vi "Shift_004.vi"() -> ()   [LabVIEW 2019]
panel:
  out "Ep(tk)":dbl[unit][](array[numeric])
  out "Et(tk)":dbl[unit][](array[numeric])
  out "Ek(tk)":dbl[unit][](array[numeric])
  out "Et":cluster{dbl[unit][], dbl[unit][]}(graph)
  out "Ep":cluster{dbl[unit][], dbl[unit][]}(graph)
  out "Ek":cluster{dbl[unit][], dbl[unit][]}(graph)
  out "Et":dbl[unit][](graph)
  out "Ep":dbl[unit][](graph)
  out "Ek":dbl[unit][](graph)
  out "a":cluster{dbl[unit][], dbl[unit][]}(graph)
  out "v":cluster{dbl[unit][], dbl[unit][]}(graph)
  out "x":cluster{dbl[unit][], dbl[unit][]}(graph)
  out "time (tk)":dbl[unit][](array[numeric])
  out "a":dbl[unit][](graph)
  out "v":dbl[unit][](graph)
  out "x":dbl[unit][](graph)
  out "x(tk)":dbl[unit][](array[numeric])
  out "v(tk)":dbl[unit][](array[numeric])
  out "a(k)":dbl[unit][](array[numeric])
  in  "M":dbl[unit]=100.0
  in  "k":dbl[unit]=1000.0
  in  "v0":dbl[unit]
  in  "x0":dbl[unit]=2.0
  in  "Dt":dbl[unit]=1e-05
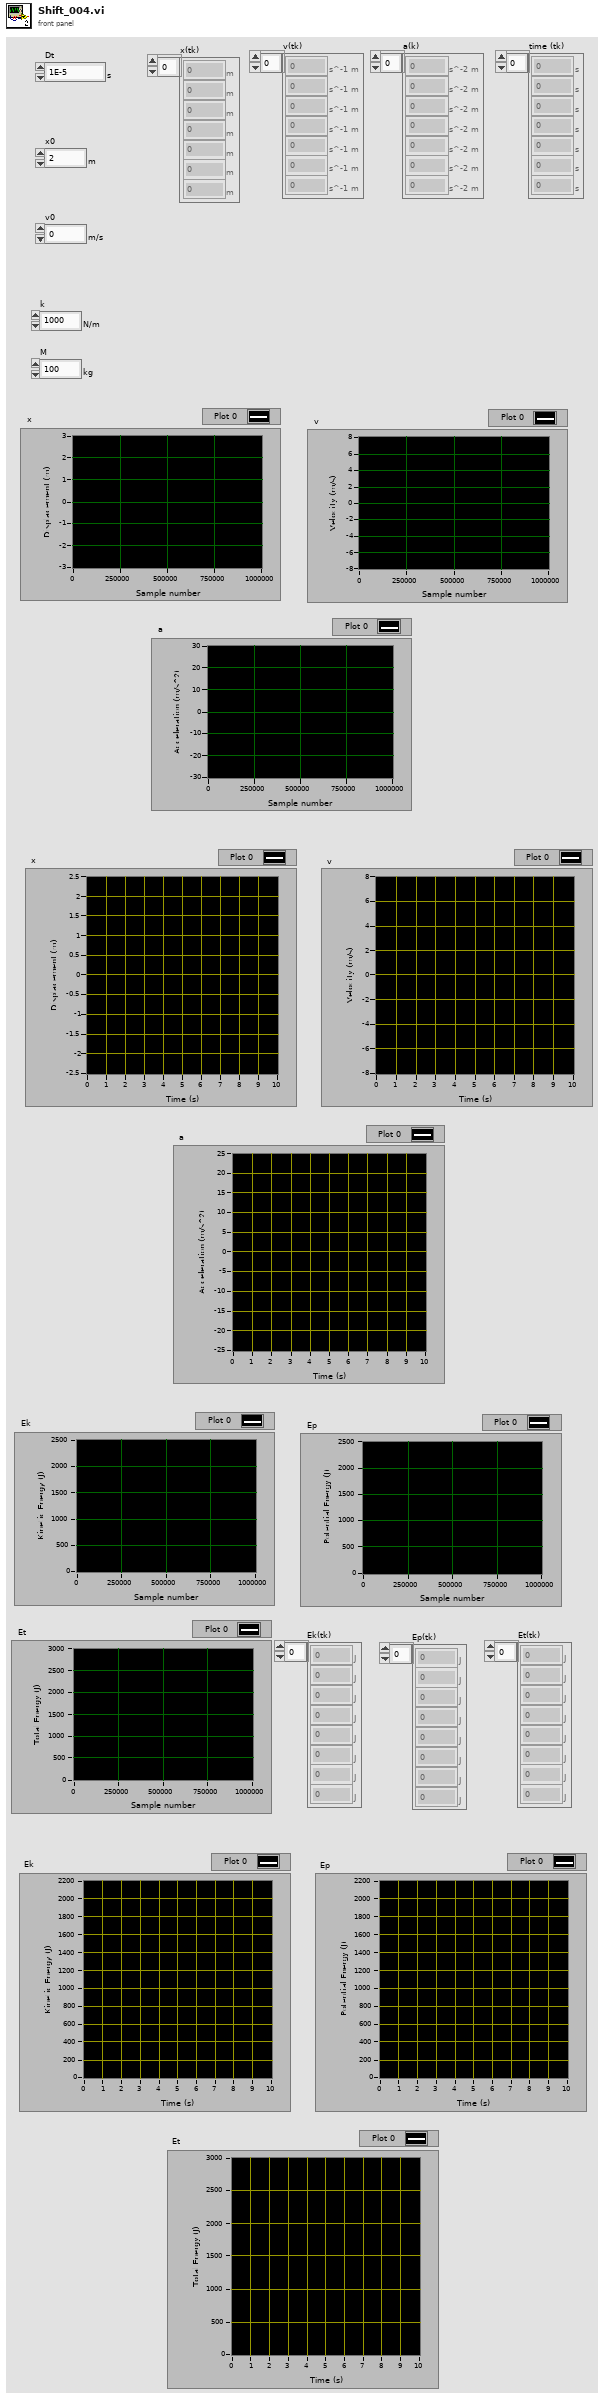
[diagram p1: front panel]
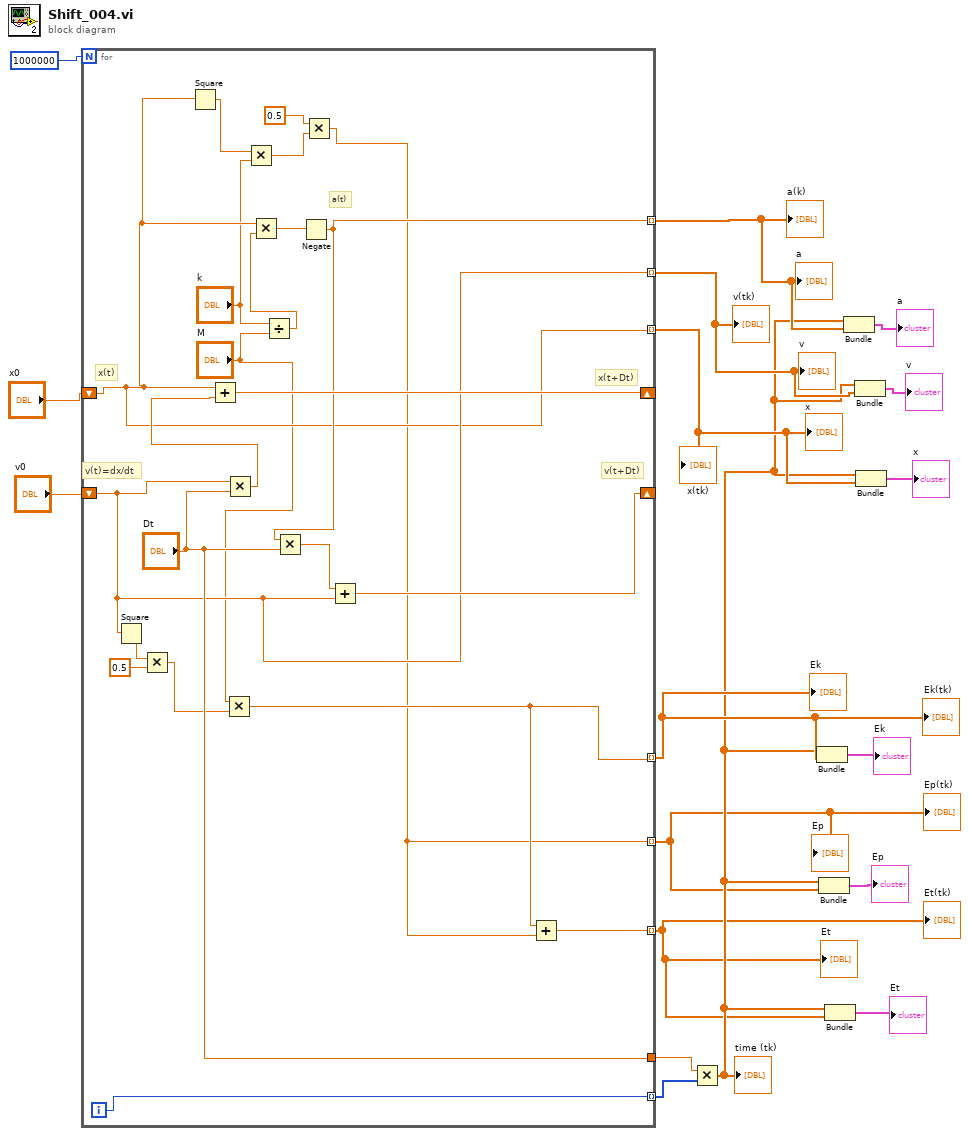
[diagram p0: block diagram]
diagram:
  n1 = for {
    N: 1000000 -> [_]
    shift-right: [w39] -> _
    shift-left: "x0" -> [w29]
    shift-right: [w36] -> _
    shift-left: "v0" -> [w31]
    tunnel: [w35] -> w10 mode=indexing
    tunnel: [w31] -> w9 mode=indexing
    tunnel: [w29] -> w8 mode=indexing
    tunnel: [w34] -> w14 mode=indexing
    tunnel: ["Dt"] -> w15
    tunnel: [w22] -> w4 mode=indexing
    tunnel: [w19] -> w1 mode=indexing
    tunnel: [w21] -> w2 mode=indexing
    i -> [w34]
    # "a(t)"
    # "v(t+Dt)"
    # "x(t+Dt)"
    # "v(t)=dx/dt"
    # "x(t)"
    n2 = Square(x=w31) -> (x^2=w30:dbl[unit])
    n3 = Multiply(x=w30, y=0.5) -> (x*y=w23:dbl[unit])
    n4 = Square(x=w29) -> (x^2=w28:dbl[unit])
    n5 = Multiply(x="M", y=w23) -> (x*y=w22:dbl[unit])
    n6 = Multiply(x=w31, y="Dt") -> (x*y=w40:dbl[unit])
    n7 = Add(x=w29, y=w40) -> (x+y=w39:dbl[unit])
    n8 = Multiply(x=w28, y="k") -> (x*y=w25:dbl[unit])
    n9 = Divide(x="k", y="M") -> (x/y=w27:dbl[unit])
    n10 = Multiply(x=w29, y=w27) -> (x*y=w38:dbl[unit])
    n11 = Negate(x=w38) -> (-x=w35:dbl[unit])
    n12 = Multiply(x=w35, y="Dt") -> (x*y=w37:dbl[unit])
    n13 = Multiply(x=0.5, y=w25) -> (x*y=w19:dbl[unit])
    n14 = Add(x=w37, y=w31) -> (x+y=w36:dbl[unit])
    n15 = Add(x=w22, y=w19) -> (x+y=w21:dbl[unit])
  }
  "a(k)" <- w10
  "v(tk)" <- w9
  "x(tk)" <- w8
  "v" <- w9
  "a" <- w10
  "x" <- w8
  "Et" <- w2
  "Ek" <- w4
  "Ep" <- w1
  "Ek(tk)" <- w4
  "Et(tk)" <- w2
  "Ep(tk)" <- w1
  n16 = Multiply(x=w15, y=w14) -> (x*y=w3:dbl[unit][])
  "time (tk)" <- w3
  n17 = Bundle(w3, w4) -> (→"Ek":cluster{dbl[unit][], dbl[unit][]})  [unwired: 1 in]
  n18 = Bundle(w3, w1) -> (→"Ep":cluster{dbl[unit][], dbl[unit][]})  [unwired: 1 in]
  n19 = Bundle(w3, w2) -> (→"Et":cluster{dbl[unit][], dbl[unit][]})  [unwired: 1 in]
  n20 = Bundle(w3, w10) -> (→"a":cluster{dbl[unit][], dbl[unit][]})  [unwired: 1 in]
  n21 = Bundle(w3, w9) -> (→"v":cluster{dbl[unit][], dbl[unit][]})  [unwired: 1 in]
  n22 = Bundle(w3, w8) -> (→"x":cluster{dbl[unit][], dbl[unit][]})  [unwired: 1 in]
